vi "Bias Setting.vi"(8 "error in (no error)":errorcluster, 9 "DC Bias Value (0.0 V)":dbl min=-40.0 max=40.0 format="%.3f", 10 "DC Bias (F:Off)":bool, 11 "VISA resource name":refnum<visa-resource-name>) -> (0 "error out":errorcluster, 3 "VISA resource name out":refnum<visa-resource-name>)   [LabVIEW 2017, in "Agilent 4194.lvlib"]
doc: "This function sets the DC bias On/Off and sets its value."
uses:
  PiezoST/Agilent 4194/Agilent 4194.lvlib
panel:
  # "On"
  # "Off"
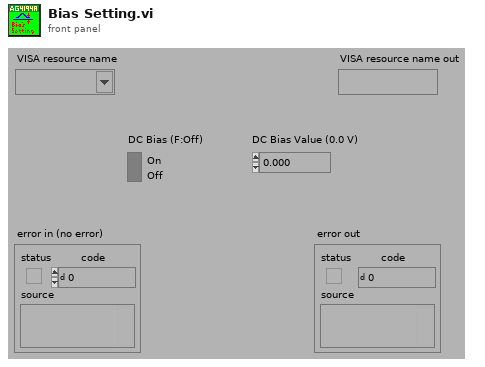
[diagram p1: front panel]
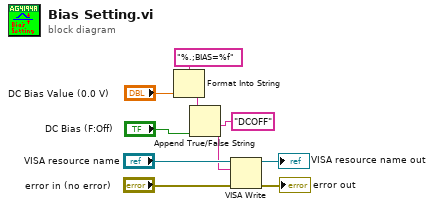
[diagram p0: block diagram]
diagram:
  n1 = Format Into String(format string="%.;BIAS=%f", "DC Bias Value (0.0 V)") -> (resulting string=w2:string)  [unwired: 2 in, 1 out]
  n2 = Append True/False String(1:"DC Bias (F:Off)", 2:"DCOFF", 3:w2) -> (0:w1:string)  [unwired: 1 in]
  n3 = VISA Write(VISA resource name="VISA resource name", write buffer=w1, error in (no error)="error in (no error)") -> (VISA resource name out=→"VISA resource name out":refnum<visa-resource-name>, error out=→"error out":errorcluster)  [unwired: 1 out]
